vi "AutomationGlobals.vi"() -> ()   [LabVIEW 2014]
panel:
  in  "StackType":dbl
  in  "LoopCount":dbl
  in  "SteerError":dbl
  out "AutoStackEnabled":bool=TRUE
  in  "AngleError":dbl=-5.2204955591712
  in  "YError":dbl=-27.0
  in  "XError":dbl=-27.0
  in  "Angle":dbl
  in  "YPos":dbl
  in  "XPos":dbl
  out "ResetGyro":bool
  out "ResetPos":bool
  in  "GantryButtons":bool[](array[boolean])
  in  "JoystickValues":dbl[](array[numeric])=[0.0, 0.0, 0.0]
  in  "ArmMaxSetpoint":dbl=110.0
  in  "Lift Max Setpoint":dbl=5156.0
  in  "Gantry Full Back Position":dbl=2638.0
  in  "Lift Setpoint Above Rails":dbl
  in  "Gantry Home Value":dbl
  in  "Lift Home Value":dbl
  in  "Barrel":bool
  in  "Number of Bins":dbl
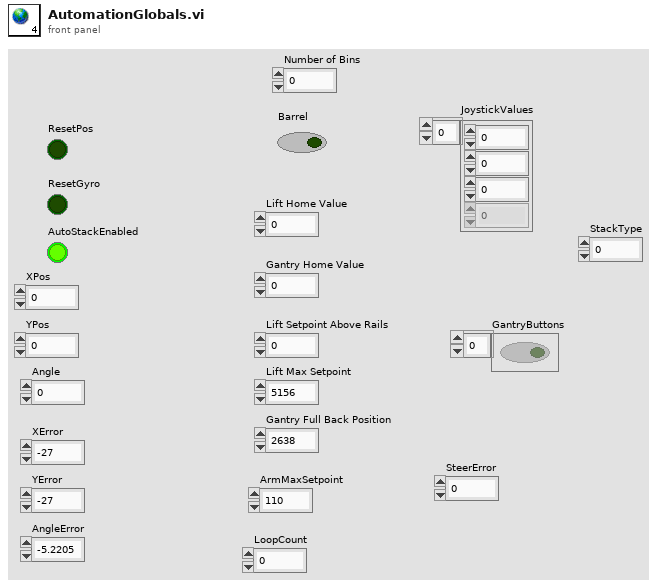
[diagram p1: front panel]
diagram:
